vi "Autorecognition of filled traps.vi"(0 "SUM Output":dbl[][](array[numeric]), 1 "Delete empty traps":bool, 2 "Manual select":bool, 3 "Manual spots trapped":i32[](array[numeric]), 5 "Store initial powers":bool, 7 "Read loaded powers":bool, 9 "Threshold":dbl format="%#_13g", 11 "Wave Reader CH 0 (MHz)":dbl[](array[numeric]) format="%#_13f", 12 "Gain CH 0 (%)":dbl[](array[numeric]), 13 "Wave Reader CH 1 (MHz)":dbl[](array[numeric]) format="%#_13f", 14 "Gain CH 1 (%)":dbl[](array[numeric])) -> (4 "Number trapped":u8, 6 "Wave Reader CH 0 (MHz) New":dbl[](array[numeric]) format="%#_13f", 8 "Gain CH 0 (%) New":dbl[](array[numeric]), 10 "Wave Reader CH 1 (MHz) New":dbl[](array[numeric]) format="%#_13f", 15 "Gain CH 1 (%) New":dbl[](array[numeric]))   [LabVIEW 2020]
panel:
  out "Spots trapped":i32[](array[numeric])
  out "Gain CH 0 (%) New 2":dbl[](array[numeric])
  out "Gain CH 1 (%) New 2":dbl[](array[numeric])
  out "Wave Reader CH 0 (MHz) New 2":dbl[](array[numeric]) format="%#_13f"
  out "Wave Reader CH 1 (MHz) New 2":dbl[](array[numeric]) format="%#_13f"
  out "Initial powers":dbl[](array[numeric])
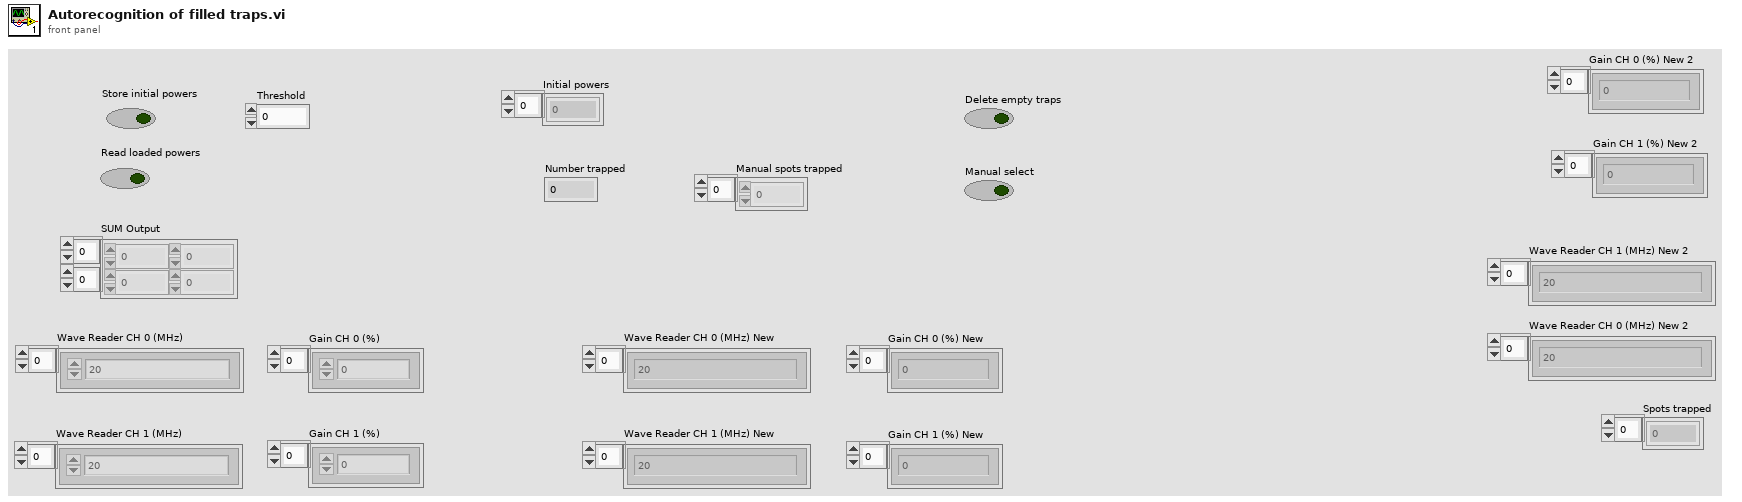
[diagram p1: front panel]
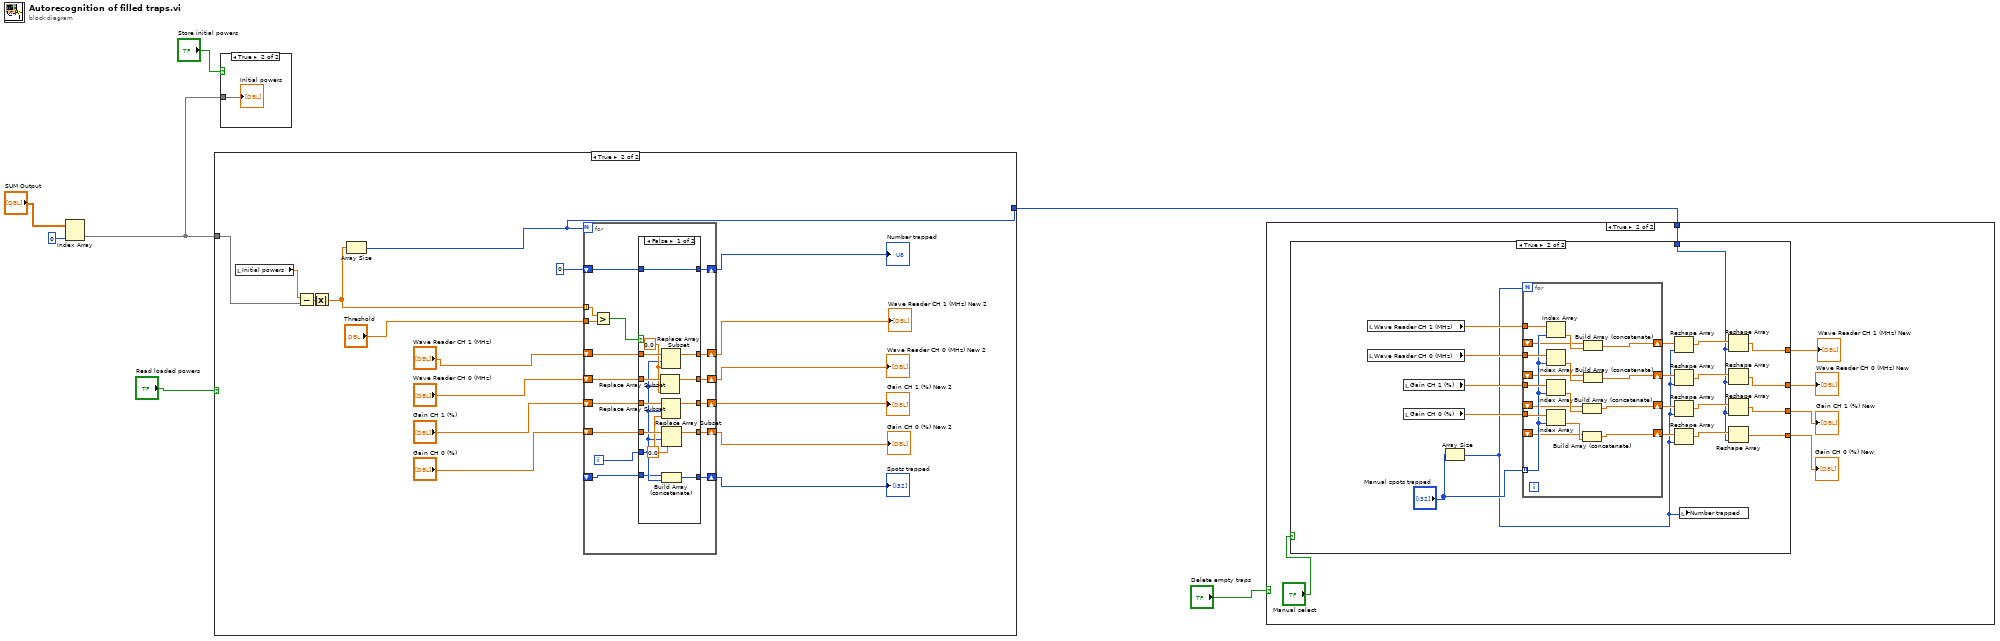
[diagram p0: block diagram]
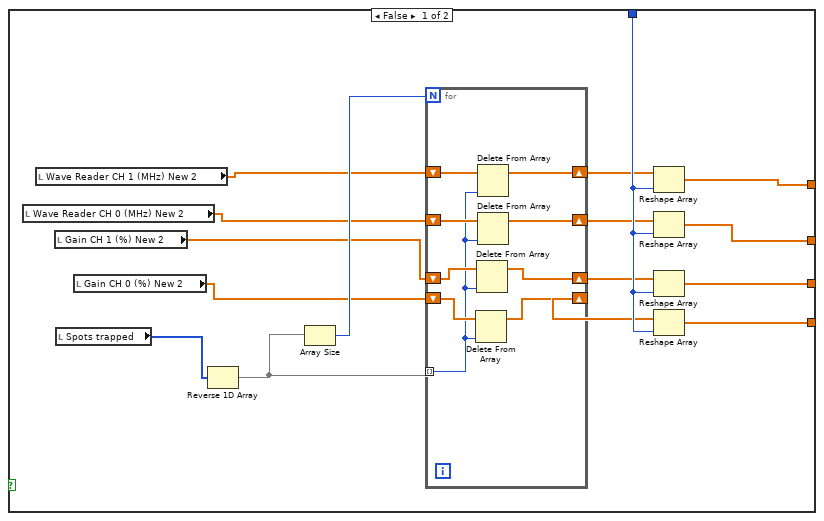
[diagram p3: hidden frame]
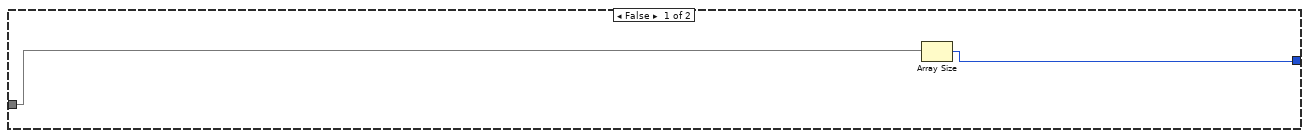
[diagram p4: hidden frame]
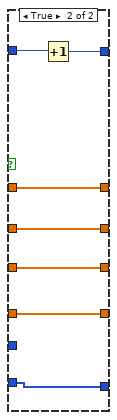
[diagram p5: hidden frame]
diagram:
  n1 = Index Array(array="SUM Output", index (col)=0) -> (element=w4:dbl[])  [unwired: 1 in]
  n2 = case shown="True" "Read loaded powers" {
    tunnel: w4 -> [w9 w26]
    tunnel: [w8 w17] -> w3
    frame False {
      n3 = Array Size(array=w9) -> (size(s)=w8:i32)
    }
    frame True {
      n4 = local read "Initial powers"() -> (w25:dbl[])
      n5 = Subtract(x=w25, y=w26) -> (x-y=w23:dbl[])
      n6 = Absolute Value(x=w23) -> (abs(x)=w22:dbl[])
      n7 = Array Size(array=w22) -> (size(s)=w17:i32)
      n8 = for {
        N: w17 -> [_]
        tunnel: w22 -> [w42] mode=indexing
        tunnel: "Threshold" -> [w41]
        shift-right: [w38] -> w11
        shift-left: "Wave Reader CH 1 (MHz)" -> [w39]
        shift-right: [w35] -> w12
        shift-left: "Wave Reader CH 0 (MHz)" -> [w36]
        shift-right: [w33] -> w13
        shift-left: "Gain CH 1 (%)" -> [w34]
        shift-right: [w31] -> w14
        shift-left: "Gain CH 0 (%)" -> [w32]
        shift-right: [w30] -> w15
        shift-left: _ -> [w29]
        shift-right: [w27] -> w10
        shift-left: u8 0 -> [w28]
        i -> [w37]
        n9 = Greater?(x=w42, y=w41) -> (0:w40:bool)
        n10 = case shown="False" w40 {
          tunnel: w39 -> [w56 w63]
          tunnel: [w55 w63] -> w38
          tunnel: w37 -> [w46 _]
          tunnel: w36 -> [w54 w62]
          tunnel: [w53 w62] -> w35
          tunnel: w34 -> [w52 w61]
          tunnel: [w51 w61] -> w33
          tunnel: w32 -> [w50 w60]
          tunnel: [w49 w60] -> w31
          tunnel: [w45 w59] -> w30
          tunnel: w29 -> [w44 w59]
          tunnel: w28 -> [w43 w58]
          tunnel: [w43 w57] -> w27
          frame False {
            w48 = 0.0 ("Frequency (Hz)")
            w47 = 0.0 ("Amplitude (V)")
            n11 = Replace Array Subset(array=w54, new element=w48, index=w46) -> (w53:dbl[])
            n12 = Replace Array Subset(array=w56, new element=w48, index=w46) -> (w55:dbl[])
            n13 = Replace Array Subset(array=w52, new element=w47, index=w46) -> (w51:dbl[])
            n14 = Replace Array Subset(array=w50, new element=w47, index=w46) -> (w49:dbl[])
            n15 = Build Array (concatenate)(w44, w46) -> (w45:i32[])
          }
          frame True {
            n16 = Increment(x=w58) -> (x+1=w57:u8)
          }
        }
      }
      "Number trapped" <- w10
      "Wave Reader CH 1 (MHz) New 2" <- w11
      "Wave Reader CH 0 (MHz) New 2" <- w12
      "Gain CH 1 (%) New 2" <- w13
      "Gain CH 0 (%) New 2" <- w14
      "Spots trapped" <- w15
    }
  }
  n17 = case shown="True" "Store initial powers" {
    tunnel: w4 -> [_ w64]
    frame False {
    }
    frame True {
      "Initial powers" <- w64
    }
  }
  n18 = case shown="True" "Delete empty traps" {
    tunnel: w3 -> [_ w70]
    frame False {
    }
    frame True {
      n19 = case shown="True" "Manual select" {
        tunnel: w70 -> [w85 w101]
        tunnel: [w80 w98] -> w69
        tunnel: [w79 w97] -> w68
        tunnel: [w78 w100] -> w67
        tunnel: [w77 w99] -> w66
        frame False {
          n20 = local read "Wave Reader CH 0 (MHz) New 2"() -> (w73:dbl[])
          n21 = local read "Wave Reader CH 1 (MHz) New 2"() -> (w72:dbl[])
          n22 = local read "Gain CH 1 (%) New 2"() -> (w74:dbl[])
          n23 = local read "Spots trapped"() -> (w71:i32[])
          n24 = local read "Gain CH 0 (%) New 2"() -> (w75:dbl[])
          n25 = Reverse 1D Array(array=w71) -> (reversed array=w86:i32[])
          n26 = Array Size(array=w86) -> (size(s)=w76:i32)
          n27 = for {
            N: w76 -> [_]
            shift-right: [w88] -> w81
            shift-left: w75 -> [w92]
            shift-right: [w89] -> w82
            shift-left: w74 -> [w93]
            shift-right: [w90] -> w83
            shift-left: w73 -> [w94]
            shift-right: [w91] -> w84
            shift-left: w72 -> [w95]
            tunnel: w86 -> [w87] mode=indexing
            n28 = Delete From Array(array=w92, index=w87) -> (array with subset deleted=w88:dbl[])  [unwired: 1 in, 1 out]
            n29 = Delete From Array(array=w93, index=w87) -> (array with subset deleted=w89:dbl[])  [unwired: 1 in, 1 out]
            n30 = Delete From Array(array=w95, index=w87) -> (array with subset deleted=w91:dbl[])  [unwired: 1 in, 1 out]
            n31 = Delete From Array(array=w94, index=w87) -> (array with subset deleted=w90:dbl[])  [unwired: 1 in, 1 out]
          }
          n32 = Reshape Array(w84, w85) -> (w78:dbl[])
          n33 = Reshape Array(w83, w85) -> (w77:dbl[])
          n34 = Reshape Array(w82, w85) -> (w80:dbl[])
          n35 = Reshape Array(w81, w85) -> (w79:dbl[])
        }
        frame True {
          n36 = local read "Wave Reader CH 1 (MHz)"() -> (w114:dbl[])
          n37 = local read "Wave Reader CH 0 (MHz)"() -> (w113:dbl[])
          n38 = local read "Gain CH 1 (%)"() -> (w112:dbl[])
          n39 = local read "Gain CH 0 (%)"() -> (w111:dbl[])
          n40 = Array Size(array="Manual spots trapped") -> (size(s)=w96:i32)
          n41 = for {
            N: w96 -> [_]
            tunnel: w114 -> [w124]
            tunnel: w113 -> [w131]
            tunnel: w112 -> [w130]
            tunnel: w111 -> [w129]
            tunnel: "Manual spots trapped" -> [w128] mode=indexing
            shift-right: [w126] -> w109
            shift-left: _ -> [w125]
            shift-right: [w120] -> w108
            shift-left: _ -> [w117]
            shift-right: [w119] -> w107
            shift-left: _ -> [w116]
            shift-right: [w118] -> w106
            shift-left: _ -> [w115]
            n42 = Index Array(array=w124, index=w128) -> (element=w127:dbl)
            n43 = Index Array(array=w131, index=w128) -> (element=w123:dbl)
            n44 = Index Array(array=w130, index=w128) -> (element=w122:dbl)
            n45 = Index Array(array=w129, index=w128) -> (element=w121:dbl)
            n46 = Build Array (concatenate)(w116, w122) -> (w119:dbl[])
            n47 = Build Array (concatenate)(w115, w121) -> (w118:dbl[])
            n48 = Build Array (concatenate)(w125, w127) -> (w126:dbl[])
            n49 = Build Array (concatenate)(w117, w123) -> (w120:dbl[])
          }
          n50 = Reshape Array(w109, w96) -> (w105:dbl[])
          n51 = Reshape Array(w108, w96) -> (w104:dbl[])
          n52 = Reshape Array(w107, w96) -> (w103:dbl[])
          n53 = Reshape Array(w106, w96) -> (w102:dbl[])
          n54 = local write "Number trapped"(w96) -> ()
          n55 = Reshape Array(w105, w101) -> (w100:dbl[])
          n56 = Reshape Array(w104, w101) -> (w99:dbl[])
          n57 = Reshape Array(w103, w101) -> (w98:dbl[])
          n58 = Reshape Array(w102, w101) -> (w97:dbl[])
        }
      }
      "Wave Reader CH 0 (MHz) New" <- w66
      "Wave Reader CH 1 (MHz) New" <- w67
      "Gain CH 0 (%) New" <- w68
      "Gain CH 1 (%) New" <- w69
    }
  }
